vi "Convert Byte Array to Float.vi"(8 "error in":errorcluster, 11 "buffer in":u8[](array[numeric])) -> (0 "error out":errorcluster, 3 "number out":sgl)   [LabVIEW 2014]
doc: "This Vi takes as input 4B (raw bit representation of float number) and convert them to float."
uses:
  Digital Filter Library.lvlib
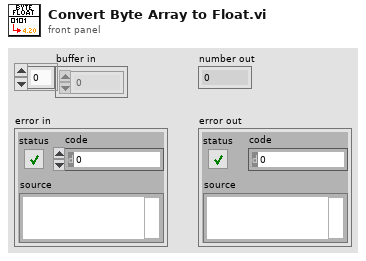
[diagram p1: front panel]
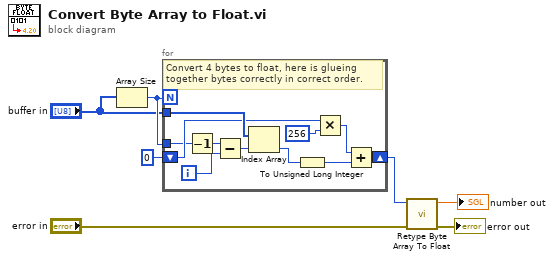
[diagram p0: block diagram]
diagram:
  n1 = Array Size(array="buffer in") -> (size(s)=w7:i32)
  n2 = for {
    N: w7 -> [_]
    tunnel: "buffer in" -> [w18]
    shift-right: [w13] -> w3
    shift-left: u32 0 ("element") -> [w17]
    tunnel: w7 -> [w12]
    i -> [w11]
    # "Convert 4 bytes to float, here is glueing together bytes correctly in correct order."
    n3 = Decrement(x=w12) -> (x-1=w10:i32)
    n4 = Subtract(x=w10, y=w11) -> (x-y=w9:i32)
    n5 = Index Array(array=w18, index=w9) -> (element=w14:u8)
    n6 = To Unsigned Long Integer(number=w14) -> (unsigned 32bit integer=w8:u32)
    n7 = Multiply(x=w17, y=u32 256) -> (x*y=w15:u32)
    n8 = Add(x=w15, y=w8) -> (x+y=w13:u32)
  }
  n9 = call "Retype Byte Array To Float.vi"("error in"="error in", "element"=w3) -> ("error out"=→"error out":errorcluster, "Numeric"=→"number out":sgl)  [unwired: 8 in]
